vi "CRIOUI.vi"() -> ()   [LabVIEW 2013, in "cRIO  node root.lvclass"]
uses:
  cRIO  node root.lvclass
  Configuration Framework/Node/NodeRef.ctl
  Configuration Framework/Node/NISE_CEF_Node.lvclass
  <vilib>/NI/AMC/Message Queue.ctl
  <vilib>/NI/AMC/Message.ctl
  <vilib>/NI/Tools/Keyed Array/KeyedArray.ctl
  Configuration Framework/Node/UserEventRef.ctl
  Configuration Framework/Controls/EventCluster.ctl
  cRIO  node root.lvclass/cRIO  node root.ctl
  <vilib>/NI/AMC/Create Single Message.vi
  <vilib>/NI/AMC/Update Message Routing Info.vi
  Configuration Framework/serializable configuration/read metadata property.vi
  <vilib>/NI/AMC/Send Message.vi
  Configuration Framework/serializable configuration/set metadata property.vi
  <vilib>/NI/AMC/AMC.lvlib
  cRIO configuration/cRIO configuration.lvclass
  <vilib>/NI/Tools/Keyed Array/Tools_KeyedArray.lvlib
  Configuration Framework/NISE_CEF_TreeControl.lvlib
panel:
  in  "user event":T1
  in  "main queue":T2
  in  "System Name":string
  in  "node ref":T3
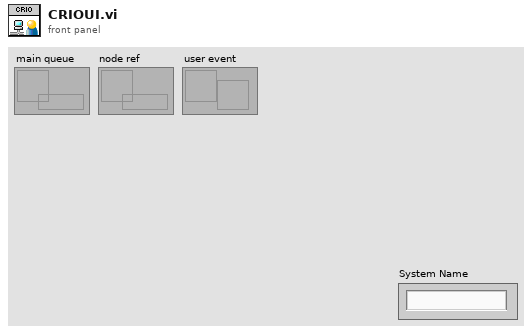
[diagram p1: front panel]
types:
  T1 = typedef "NISE_CEF_Node.lvclass/UserEventRef.ctl" = refnum<user-event>
  T2 = typedef "AMC.lvlib/Message Queue.ctl" = refnum<queue>
  T3 = typedef "NISE_CEF_Node.lvclass/NodeRef.ctl" = refnum<data-value>
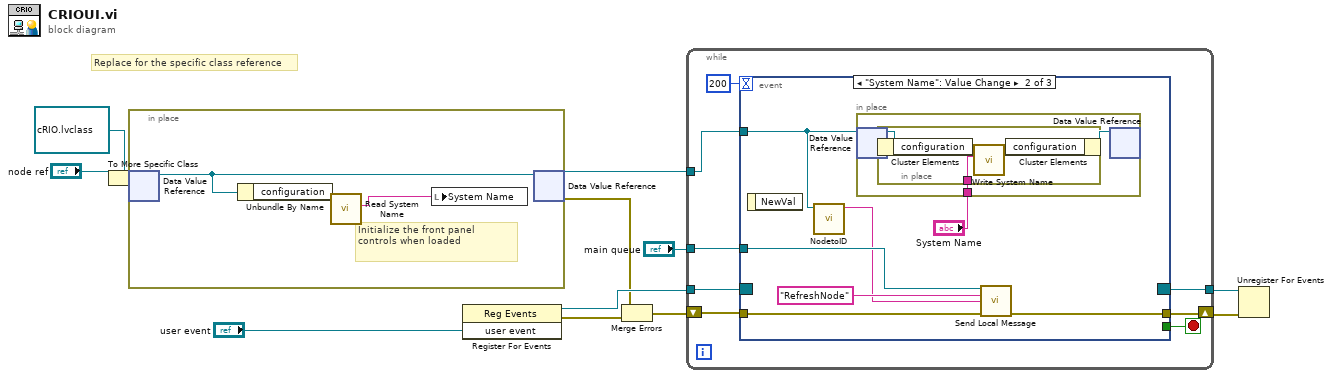
[diagram p0: block diagram]
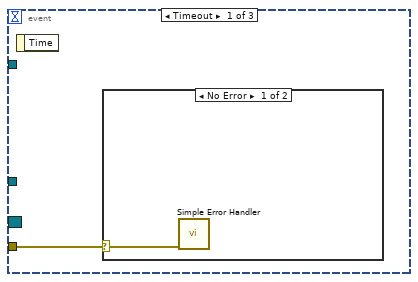
[diagram p2: hidden frame]
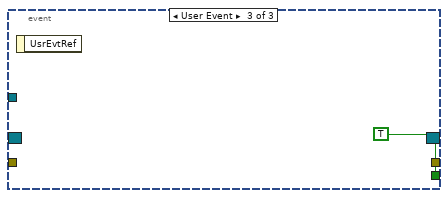
[diagram p4: hidden frame]
diagram:
  # "Replace for the specific class reference"
  n1 = To More Specific Class(target class=refnum<data-value> refnum ("data value reference"), reference="node ref") -> (specific class reference=w5:refnum<data-value>)  [unwired: 1 in, 1 out]
  n2 = in-place {
    # "Initialize the front panel controls when loaded"
    n3 = in-place-dvr #1(w5) -> (w14:refnum<class "cRIO  node root.lvclass">)  [unwired: 1 out]
    n4 = Unbundle By Name(w14) -> ("configuration"=w13:refnum<class "cRIO configuration.lvclass">)
    n5 = call "Read System Name.vi"("crio configuration in"=w13) -> ("System Name"=w15:string)  [unwired: 8 in, 2 out]
    n6 = local write "System Name"(w15) -> ()
    n7 = in-place-dvr #1(w14) -> (w12:refnum<data-value>, w2:errorcluster)
  }
  n8 = register-events("user event") -> (reference out=w9:refnum<event-registration>, error out=w3:errorcluster)  [unwired: 2 in]
  n9 = Merge Errors(w2, w3) -> (w1:errorcluster)
  n10 = while {
    tunnel: w12 -> [w23]
    tunnel: "main queue" -> [w22]
    tunnel: w9 -> [w20]
    tunnel: [w19] -> w8
    shift-right: [w17] -> w7
    shift-left: w1 -> [w16]
    stop <- w18 stop-if-true
    n11 = event shown="[1] \"System Name\": Value Change" {
      selector: w20 -> [_ _ _]
      dyn-events: [_ _ _] -> w19
      timeout: 200 -> [_ _ _]
      tunnel: w23 -> [_ w30 _]
      tunnel: w22 -> [_ w31 _]
      tunnel: [_ _ TRUE] -> w18
      tunnel: [_ w28 _] -> w17
      tunnel: w16 -> [w24 w27 _]
      event Timeout {
        n12 = event-data() -> ()  [unwired: 1 in, 1 out]
        n13 = case shown="No Error" w24 {
          selector: w24 -> [w25 _]
          frame No Error {
            n14 = call <vilib>:"Simple Error Handler.vi"("error in (no error)"=w25) -> ()  [unwired: 4 in, 5 out]
          }
          frame Error {
          }
        }
      }
      event "System Name": Value Change {
        n15 = event-data() -> ()  [unwired: 1 in, 1 out]
        n16 = call "NodetoID.vi"("node ref"=w30) -> ("ID"=w29:string)  [unwired: 9 in, 1 out]
        n17 = in-place {
          in-place-border: "System Name" -> [w33]
          n18 = in-place-dvr #2(w30) -> (w35:refnum<class "cRIO  node root.lvclass">)  [unwired: 1 out]
          n19 = in-place {
            in-place-border: w33 -> [w36]
            n20 = in-place-cluster #3(w35) -> ("configuration"=w38:refnum<class "cRIO configuration.lvclass">)
            n21 = call "Write System Name.vi"("System Name"=w36, "crio configuration in"=w38) -> ("crio configuration out"=w37:refnum<class "cRIO configuration.lvclass">)  [unwired: 8 in, 1 out]
            n22 = in-place-cluster #3("configuration"=w37) -> (w34:refnum<class "cRIO  node root.lvclass">)
          }
          n23 = in-place-dvr #2(w34) -> ()  [unwired: 2 out]
        }
        n24 = call <vilib>:"Send Local Message.vi"("message queue in"=w31, "message name"="RefreshNode" ("Message Name"), "message value"=w29, "error in"=w27) -> ("error out"=w28:errorcluster)  [unwired: 9 in, 2 out]
      }
      event User Event {
        n25 = event-data() -> ()  [unwired: 1 in, 1 out]
      }
    }
  }
  n26 = Unregister For Events(event registration refnum=w8, error in=w7) -> ()  [unwired: 1 out]
